vi "Enqueue Array of Strings.vi"(8 "error in (no error)":errorcluster, 10 "Array":string[](array[string]), 11 "queue":refnum<queue>) -> (0 "error out":errorcluster, 3 "queue out":refnum<queue>)   [LabVIEW 2018]
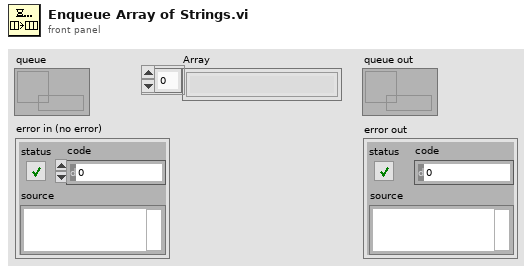
[diagram p1: front panel]
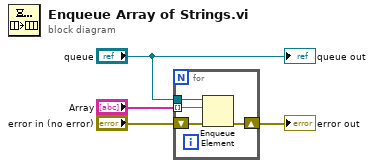
[diagram p0: block diagram]
diagram:
  n1 = for {
    tunnel: "queue" -> [w8]
    tunnel: "Array" -> [w5] mode=indexing
    shift-right: [w6] -> w4
    shift-left: "error in (no error)" -> [w7]
    n2 = Enqueue Element(queue=w8, element=w5, error in (no error)=w7) -> (error out=w6:errorcluster)  [unwired: 1 in, 2 out]
  }
  "error out" <- w4
  "queue out" <- "queue"
